vi "Connect.vi"(8 "error in (no error)":errorcluster, 11 "GEN40-38-LAN in":refnum<class "GEN40-38-LAN.lvclass">) -> (0 "error out":errorcluster, 3 "GEN40-38-LAN out":refnum<class "GEN40-38-LAN.lvclass">)   [LabVIEW 2018, in "GEN40-38-LAN.lvlib" / "GEN40-38-LAN.lvclass"]
uses:
  GEN40-38-LAN.lvclass
  GEN40-38-LAN.lvclass/GEN40-38-LAN.ctl
  PPLs/Power Supply/Parent/Power_Supply.lvlibp/Power Supply.lvclass
  C:/Projects/LabVIEW/PPLs/Power Supply/Parent/Power_Supply.lvlibp/Power Supply.lvclass
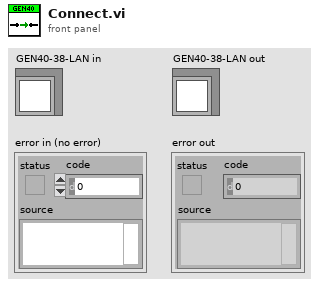
[diagram p1: front panel]
types:
  T1 = typedef "GEN40-38-LAN.lvlib/GEN40-38-LAN.lvclass/Identification.ctl" = cluster{"Manufacturer":string, "Model":string, "Serial Number":string, "Revisions":string}
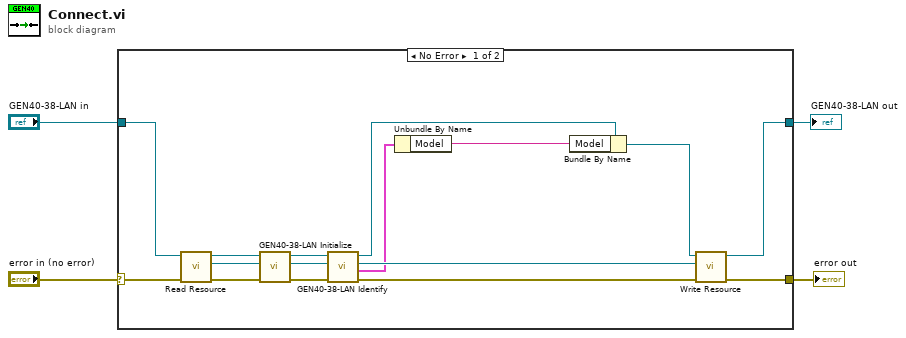
[diagram p0: block diagram]
diagram:
  n1 = case shown="No Error" "error in (no error)" {
    selector: "error in (no error)" -> [w8 w21]
    tunnel: [w19 w21] -> w3
    tunnel: [w18 w20] -> w1
    tunnel: "GEN40-38-LAN in" -> [w9 w20]
    frame No Error {
      n2 = call "Read Resource.vi"("error in"=w8, "Power Supply in"=w9) -> ("error out"=w7:errorcluster, "Resource"=w5:refnum<visa-resource-name>, "Power Supply out"=w6:refnum<class "GEN40-38-LAN.lvclass">)  [unwired: 7 in]
      n3 = call "GEN40-38-LAN Initialize.vi"("error in (no error)"=w7, "VISA resource name"=w5, "GEN40-38-LAN in"=w6) -> ("error out"=w15:errorcluster, "VISA resource name out"=w16:refnum<visa-resource-name>, "GEN40-38-LAN out"=w17:refnum<class "GEN40-38-LAN.lvclass">)  [unwired: 6 in]
      n4 = call "GEN40-38-LAN Identify.vi"("error in (no error)"=w15, "VISA resource name out"=w16, "GEN40-38-LAN in"=w17) -> ("error out"=w11:errorcluster, "Identification"=w14:T1, "GEN40-38-LAN out"=w13:refnum<class "GEN40-38-LAN.lvclass">)  [unwired: 6 in]
      n5 = Unbundle By Name(w14) -> ("Model"=w10:string)
      n6 = Bundle By Name(cluster=w13, "Model"=w10) -> (w12:refnum<class "GEN40-38-LAN.lvclass">)
      n7 = call "Write Resource.vi"("error in"=w11, "Resource"=w16, "Power Supply in"=w12) -> ("error out"=w19:errorcluster, "Power Supply out"=w18:refnum<class "GEN40-38-LAN.lvclass">)  [unwired: 7 in]
    }
    frame Error {
    }
  }
  "error out" <- w3
  "GEN40-38-LAN out" <- w1
